vi "Clear_broken_frames_2_v16_171213.vi"(11 "Input  data 2D array":dbl[][](array[numeric])) -> (1 "Cleaned array":dbl[][](array[numeric]), 2 "Errors array":dbl[][](array[numeric]), 3 "Number of errors":i32)   [LabVIEW 2018]
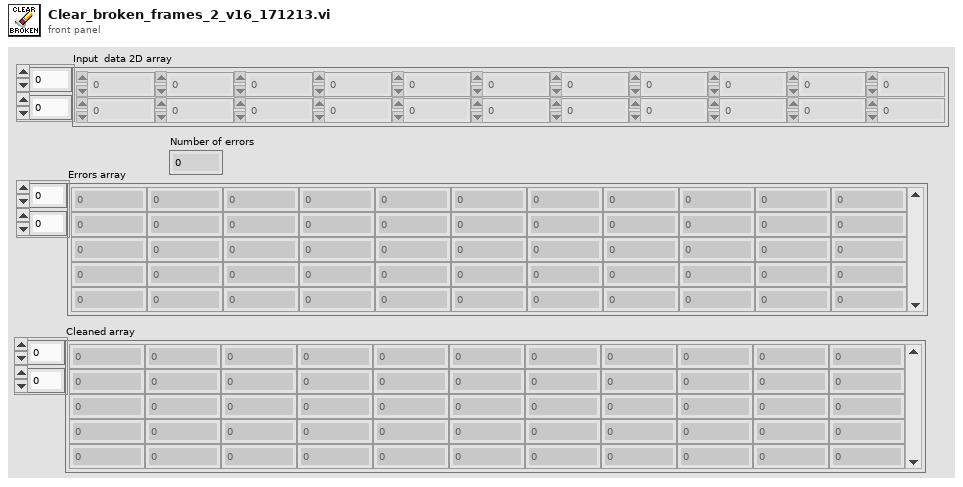
[diagram p1: front panel]
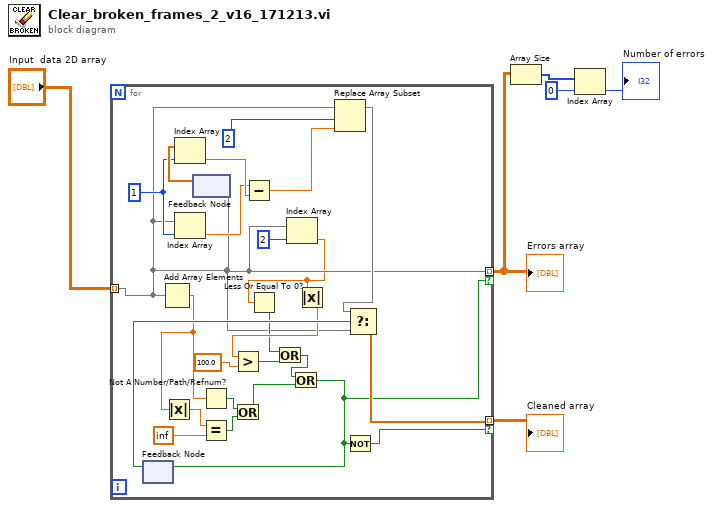
[diagram p0: block diagram]
diagram:
  n1 = for {
    tunnel: "Input  data 2D array" -> [w9] mode=indexing
    tunnel: [w9] -> w3 mode=indexing if=w17
    tunnel: [w30] -> w2 mode=indexing if=w31
    w25 = 1 ("index")
    n2 = feedback #1() -> (w29:bool)  [unwired: 1 in]
    n3 = Add Array Elements(numeric array=w9) -> (sum=w19:dbl)
    n4 = Absolute Value(x=w19) -> (abs(x)=w18:dbl)
    n5 = Index Array(array=w9, index=w25) -> (element=w23:dbl)
    n6 = feedback #2() -> (w28:dbl[])  [unwired: 1 in]
    n7 = Index Array(array=w28, index=w25) -> (element=w24:dbl)
    n8 = feedback-in #2(w9) -> ()
    n9 = Not A Number/Path/Refnum?(number/path/refnum=w19) -> (NaN/Path/Refnum?=w22:bool)
    n10 = Equal?(x=w18, y=inf) -> (x = y?=w21:bool)
    n11 = Or(x=w22, y=w21) -> (x .or. y?=w16:bool)
    n12 = Subtract(x=w23, y=w24) -> (x-y=w11:dbl)
    n13 = Index Array(array=w9, index=2) -> (element=w7:dbl)
    n14 = Less Or Equal To 0?(x=w7) -> (x <= 0?=w10:bool)
    n15 = Absolute Value(x=w7) -> (abs(x)=w14:dbl)
    n16 = Greater?(x=w14, y=100.0) -> (0:w13:bool)
    n17 = Or(x=w10, y=w13) -> (x .or. y?=w12:bool)
    n18 = Or(x=w12, y=w16) -> (x .or. y?=w17:bool)
    n19 = feedback-in #1(w17) -> ()
    n20 = Replace Array Subset(array=w9, new element=w11, index=2) -> (w26:dbl[])
    n21 = Not(x=w17) -> (.not. x?=w31:bool)
    n22 = Select(t=w26, s=w29, f=w9) -> (s? t:f=w30:dbl[])
  }
  "Errors array" <- w3
  "Cleaned array" <- w2
  n23 = Array Size(array=w3) -> (size(s)=w4:i32[])
  n24 = Index Array(array=w4, index=0) -> (element=→"Number of errors":i32)
